vi "beam cup control - old.vi"() -> ()   [LabVIEW 2016, in "Top Level.lvlib"]
doc: "This vi is used to control the cups and apertures in the ams beamline."
uses:
  Top Level.lvlib
panel:
  in  "Which Beamline":string(combo)="R45"
  out "R45 detector cup":string="OUT"
  out "R45 detector aperture":string="IN"
  out "R45 switch image cup":string="IN"
  out "R45 switch aperture":string="OUT"
  in  "R30 detector ap":bool=TRUE
  out "R30 detector aperture":string="IN"
  out "R30 Detector cup rd":string="OUT"
  out "R30 switch aperture":string="IN"
  in  "R30 Image ap":bool=TRUE
  out "R30 switch image cup":string="OUT"
  out "analyze image cup rd":string="OUT"
  out "tank exit cup  rd":string="OUT"
  out "tank entrance cup  rd":string="OUT"
  out "low energy cup":string="OUT"
  out "injector image aperture":string="IN"
  out "injector cup":string="OUT"
  in  "r45 det cup":bool
  in  "R45  det ap":bool
  in  "r45 switch image cup":bool=TRUE
  in  "R45 #1 ap":bool
  out "Terminal Voltage":dbl=8.333384070396422 format="%#_4g"
  in  "R30 det cup":bool
  in  "Switch magnet cup":bool
  in  "Analyze image cup":bool
  in  "Tank exit cup":bool
  in  "Tank Entrance cup":bool
  in  "Low end waist  cup":bool=TRUE
  in  "Low end waist ap":bool
  in  "INJ Image ap":bool
  in  "Inj Image cup":bool
  out "date/time string":string="3/16/2012  11:07 AM"
  out "Error out":errorcluster
  in  "stop":bool
  # "Faraday cup Controls"
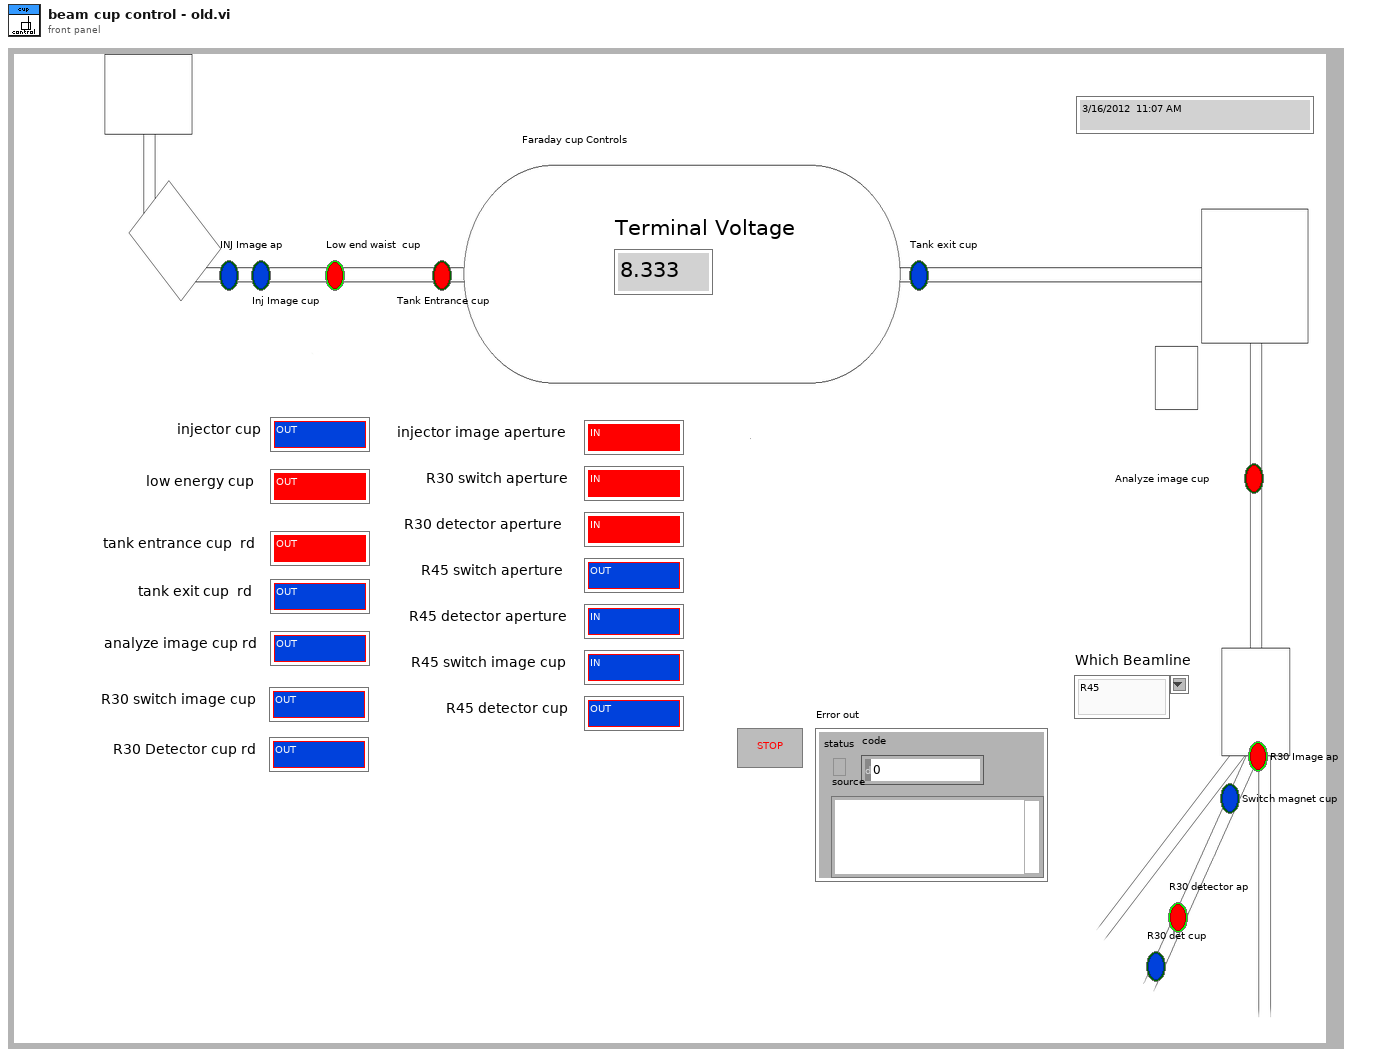
[diagram p1: front panel]
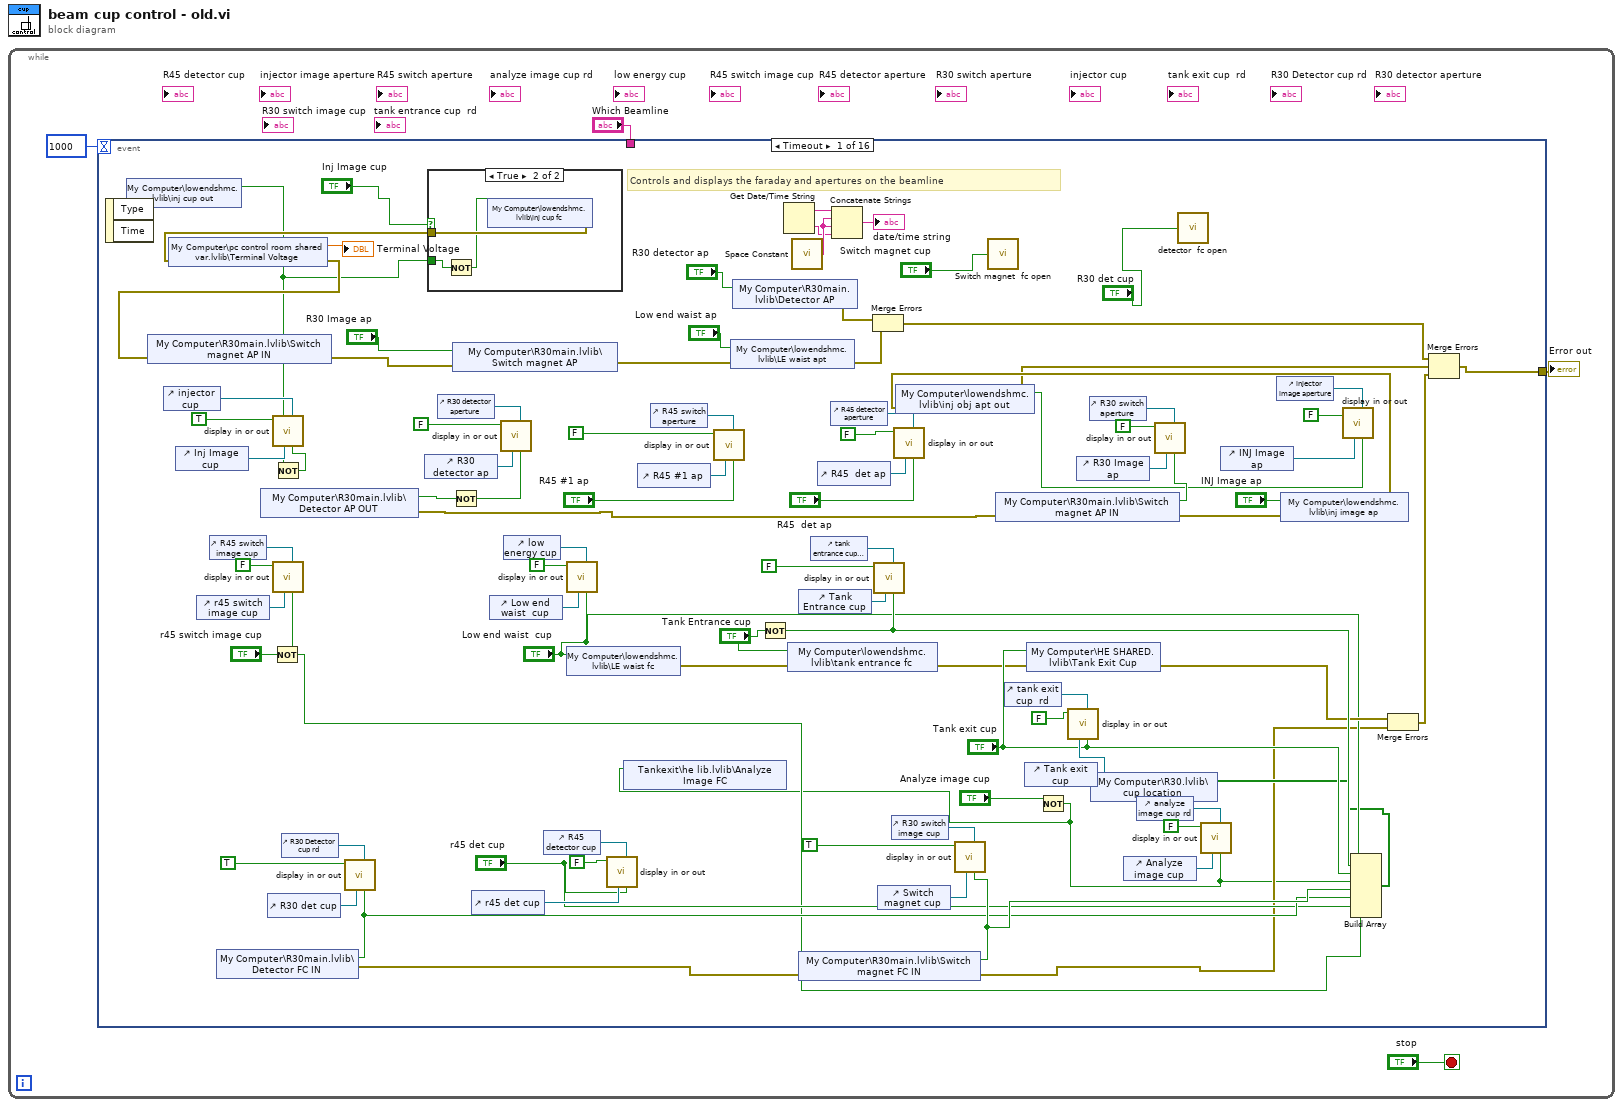
[diagram p0: block diagram]
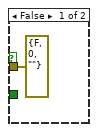
[diagram p2: hidden frame]
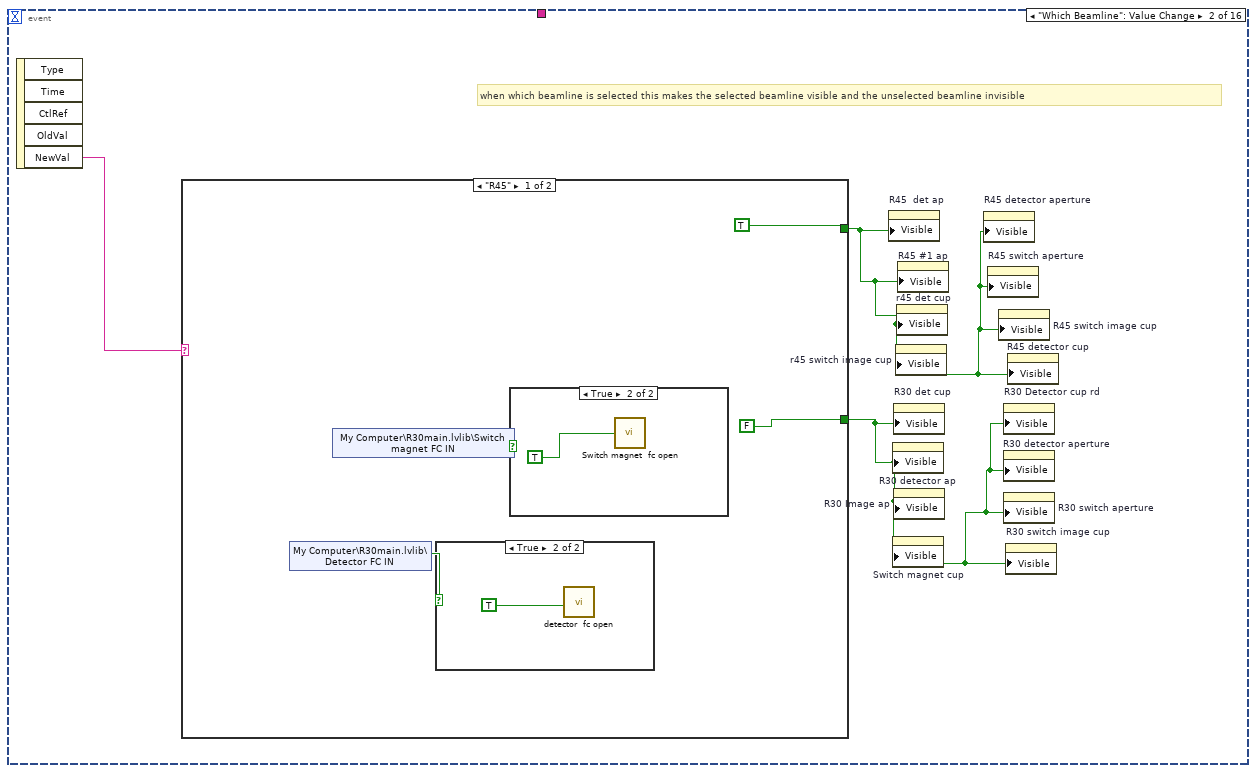
[diagram p3: hidden frame]
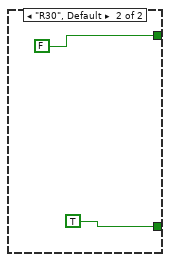
[diagram p6: hidden frame]
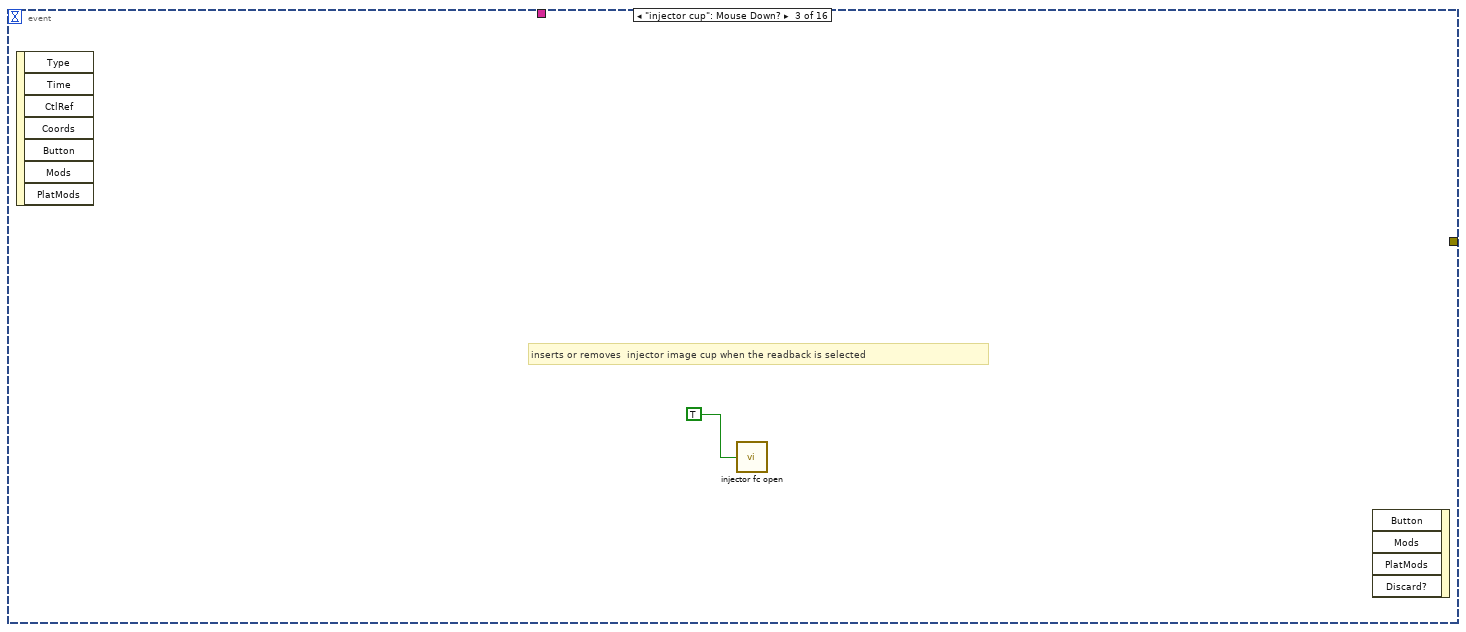
[diagram p7: hidden frame]
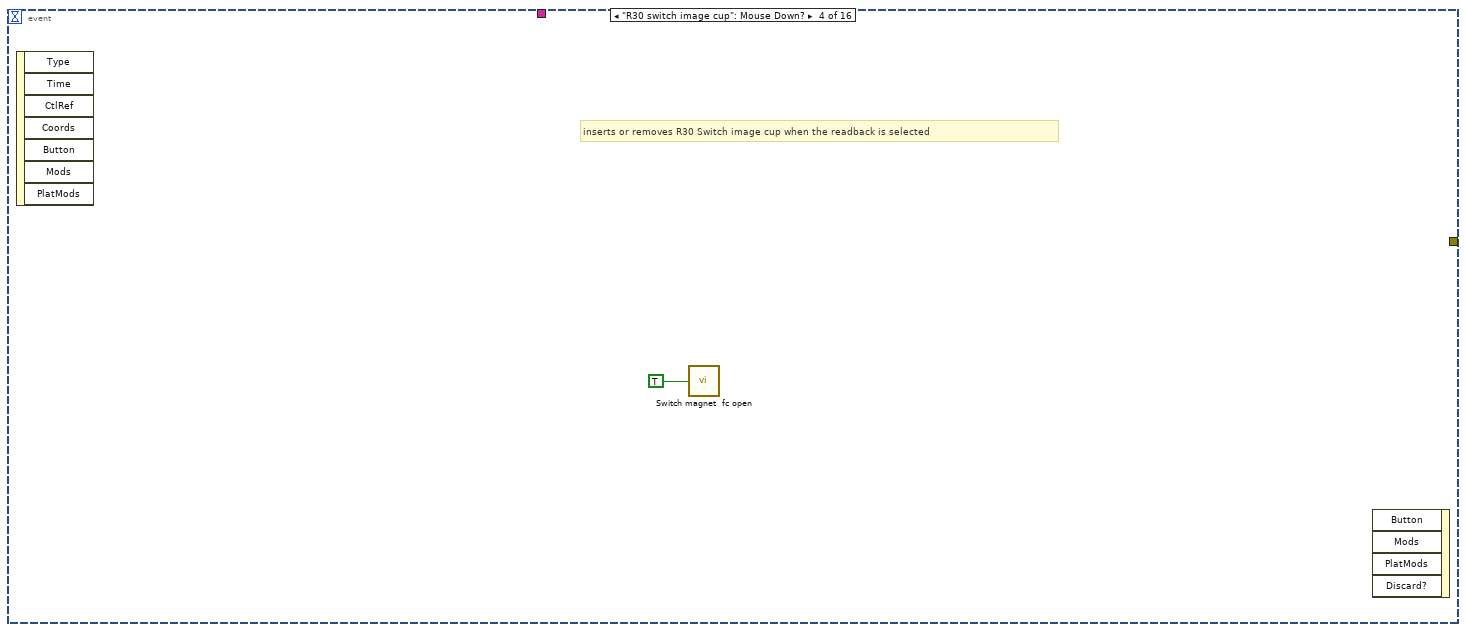
[diagram p8: hidden frame]
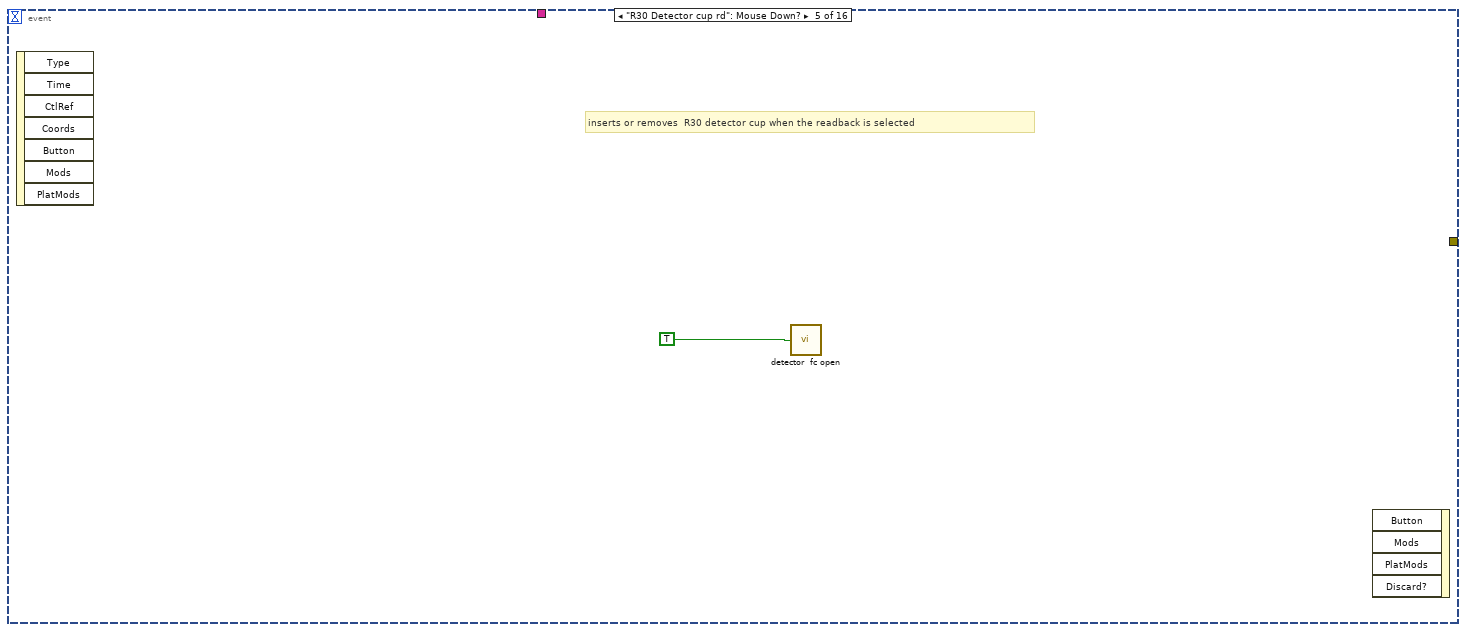
[diagram p9: hidden frame]
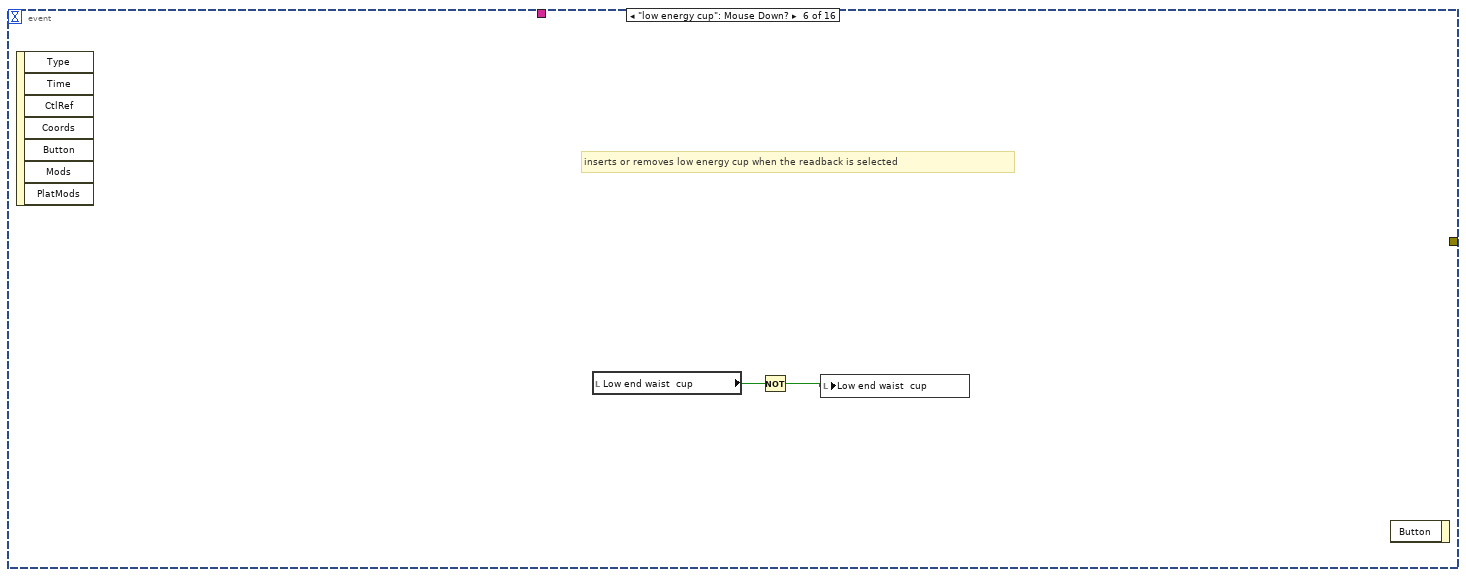
[diagram p10: hidden frame]
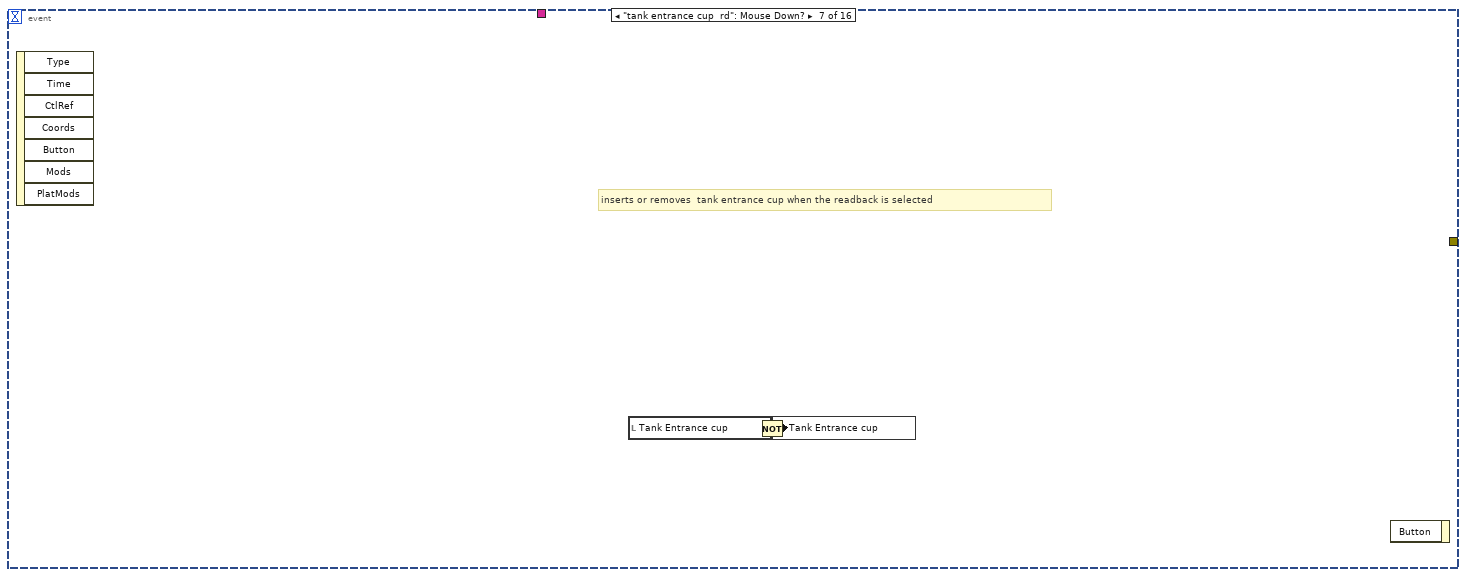
[diagram p11: hidden frame]
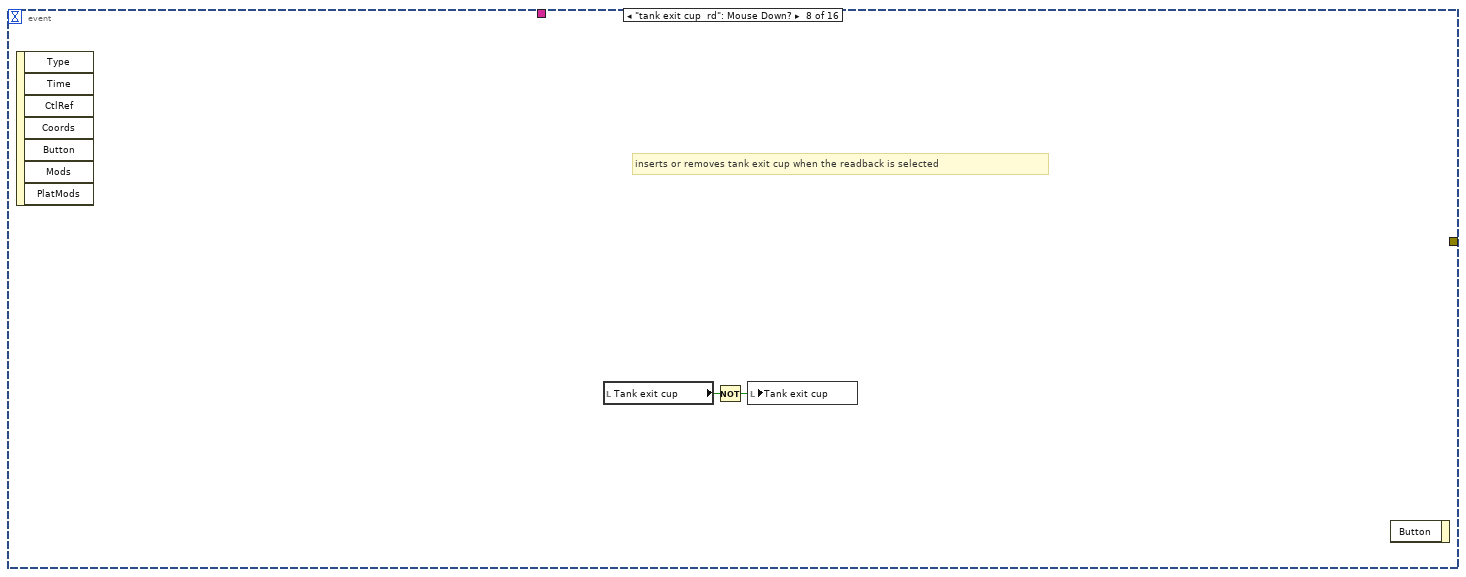
[diagram p12: hidden frame]
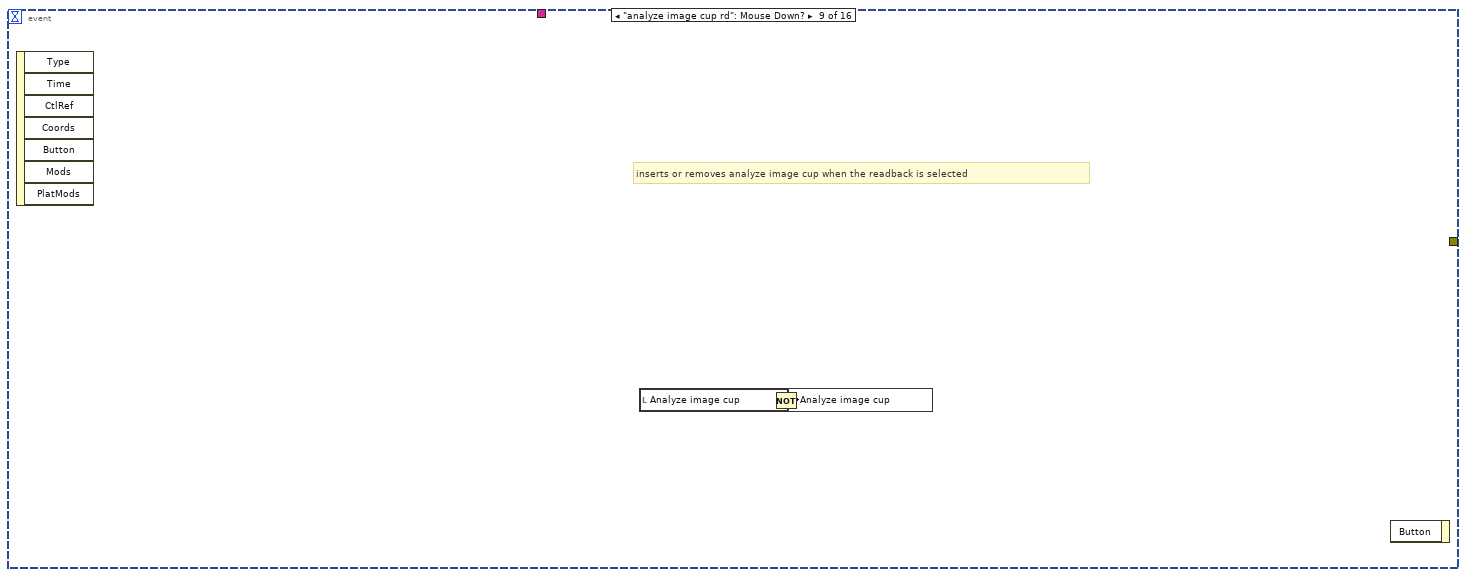
[diagram p13: hidden frame]
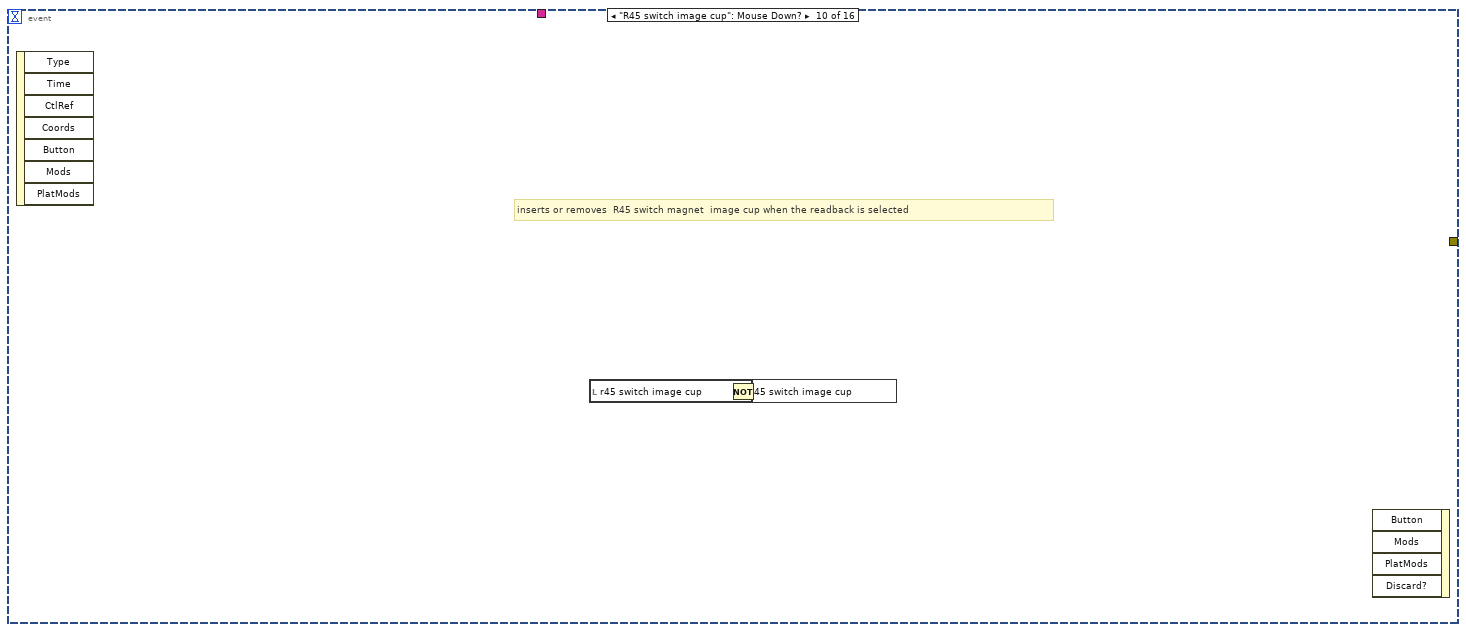
[diagram p14: hidden frame]
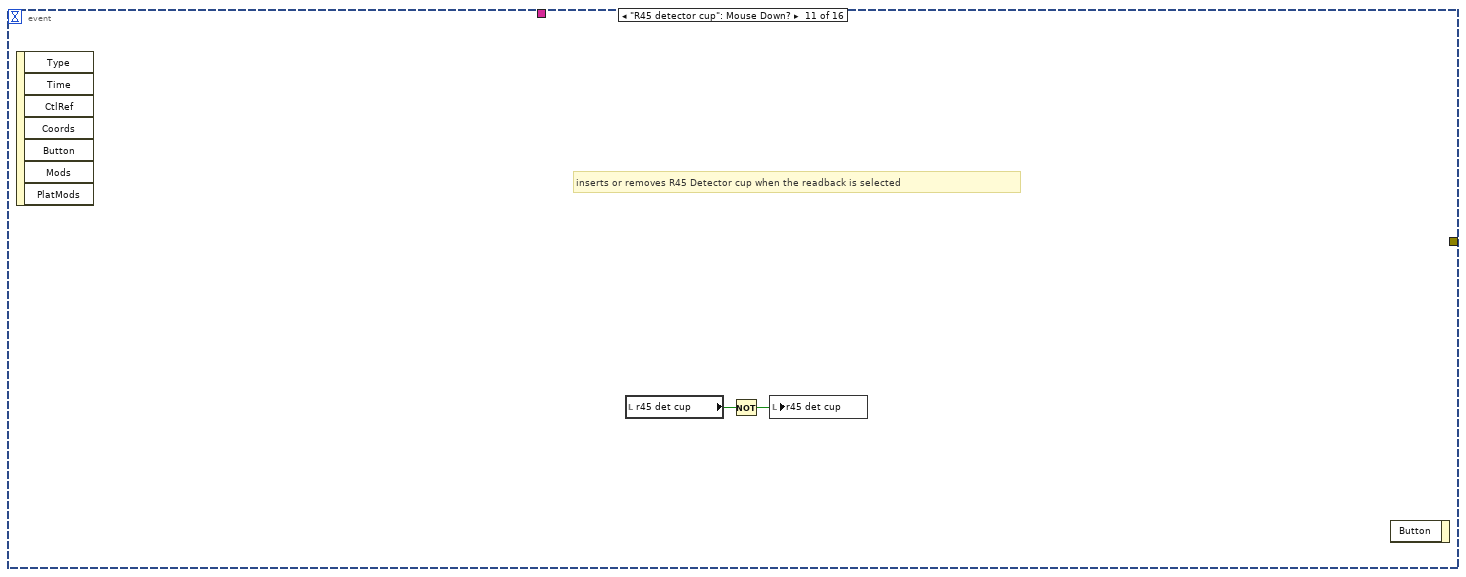
[diagram p15: hidden frame]
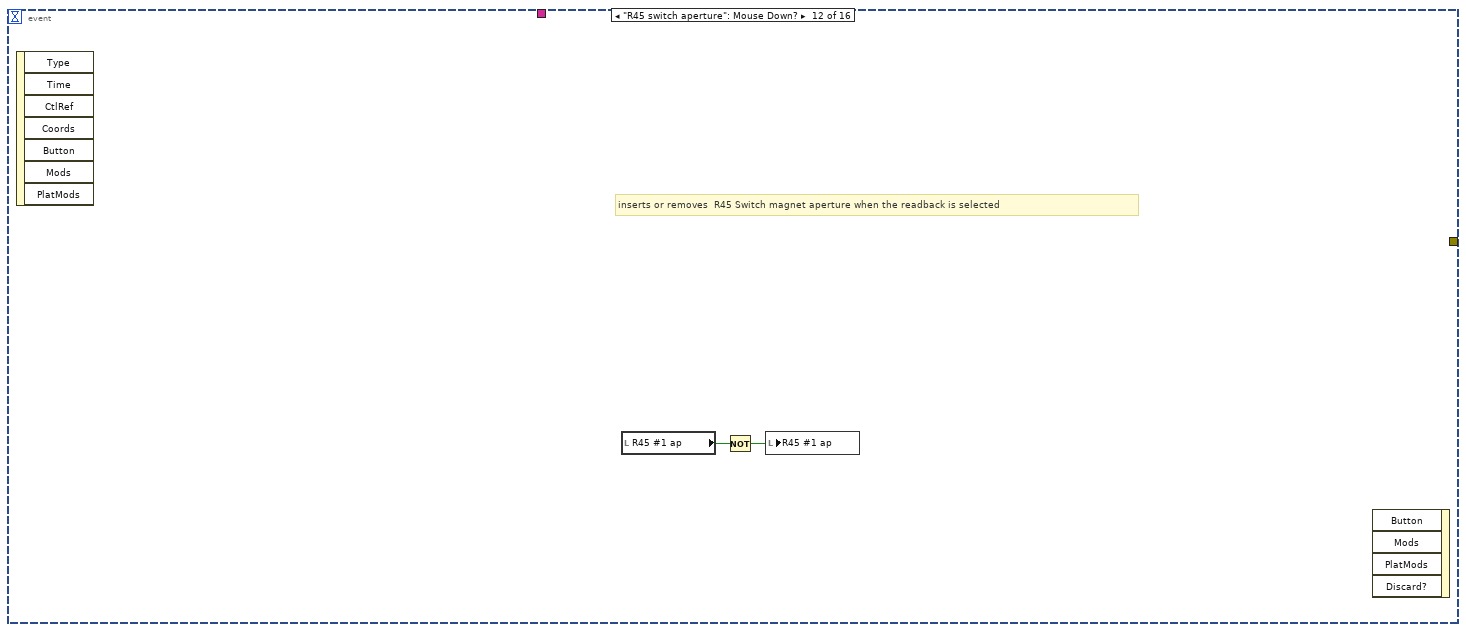
[diagram p16: hidden frame]
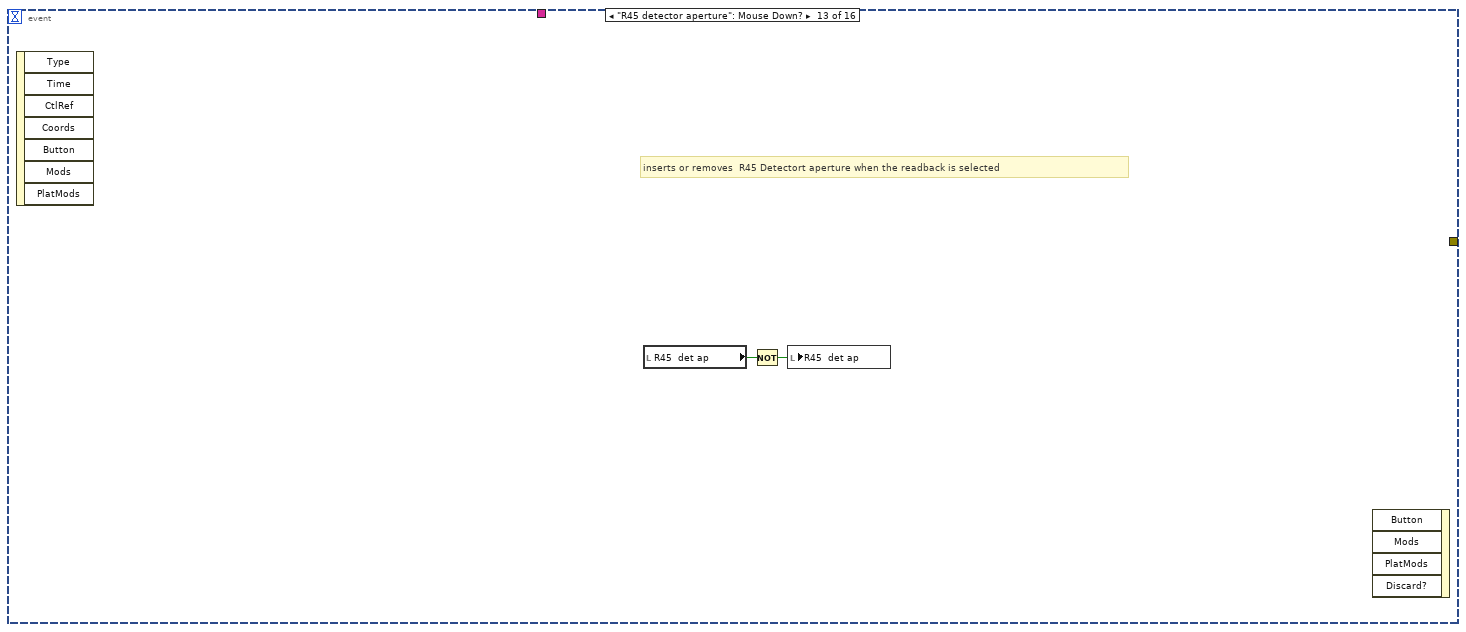
[diagram p17: hidden frame]
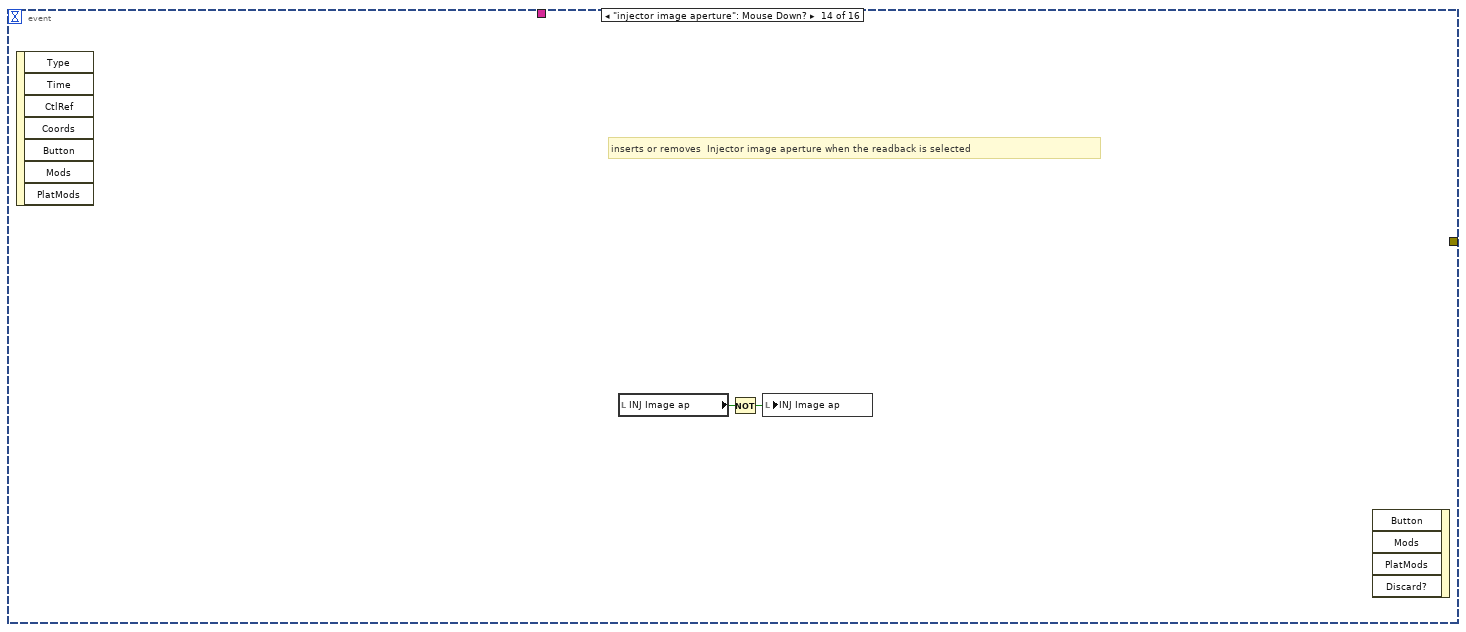
[diagram p18: hidden frame]
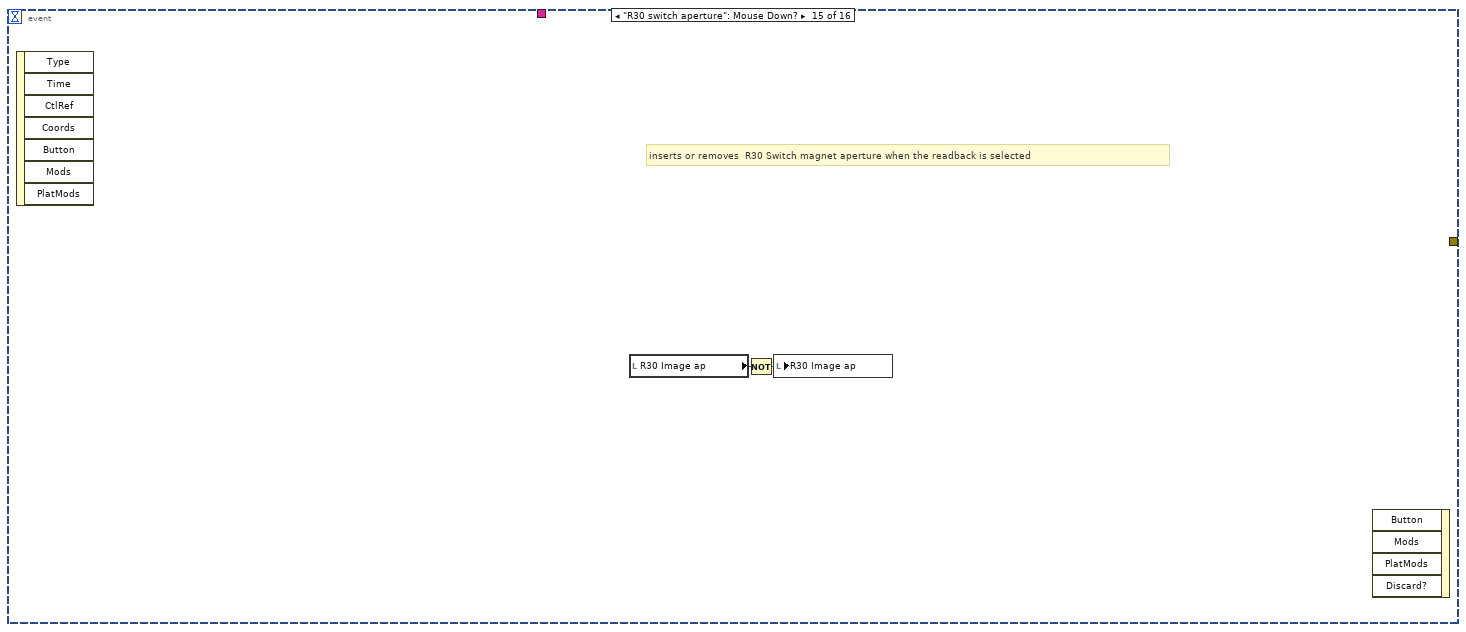
[diagram p19: hidden frame]
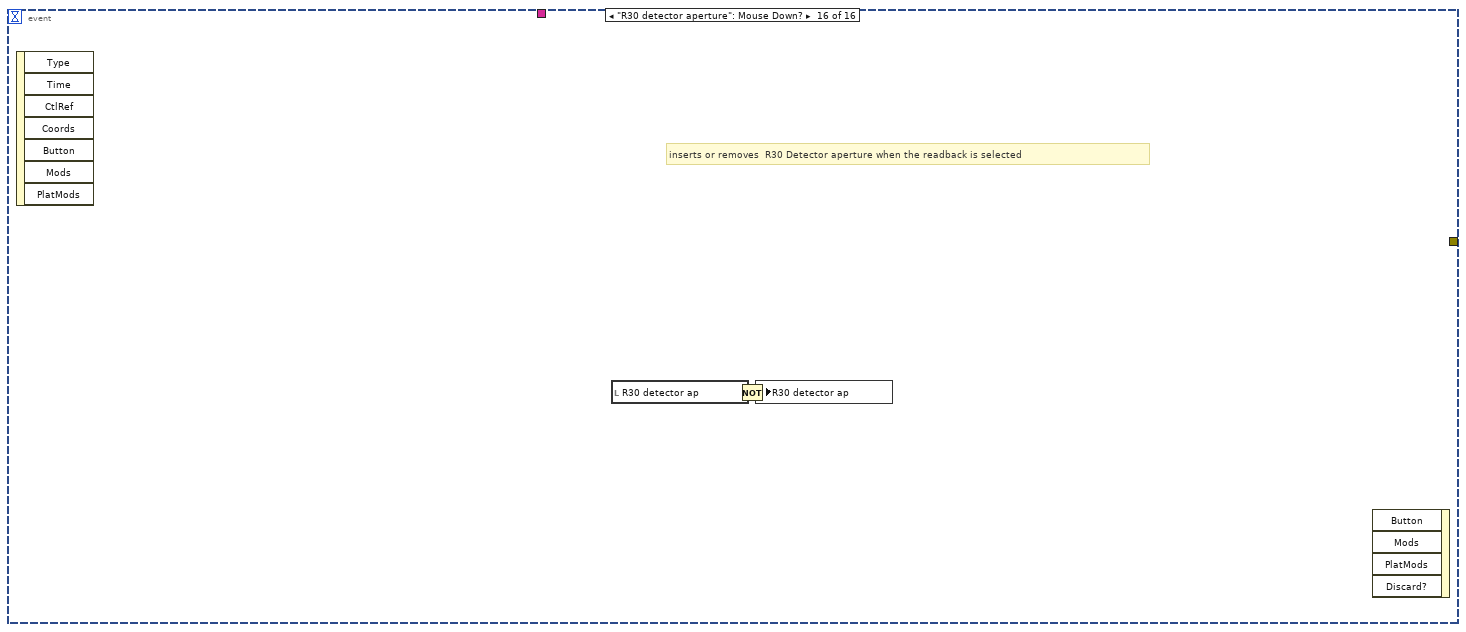
[diagram p20: hidden frame]
diagram:
  n1 = while {
    stop <- "stop" stop-if-true
    n2 = event shown="[0] Timeout" {
      selector: _ -> [_ _ _ _ _ _ _ _ _ _ _ _ _ _ _ _]
      dyn-events: _ -> [_ _ _ _ _ _ _ _ _ _ _ _ _ _ _ _]
      timeout: 1000 -> [_ _ _ _ _ _ _ _ _ _ _ _ _ _ _ _]
      tunnel: [w24 _ _ _ _ _ _ _ _ _ _ _ _ _ _ _] -> w2
      tunnel: "Which Beamline" -> [_ _ _ _ _ _ _ _ _ _ _ _ _ _ _ _]
      event Timeout {
        # "Controls and displays the faraday and apertures on the beamline"
        n3 = event-data() -> ()  [unwired: 1 in, 2 out]
        n4 = shared-variable "My Computer\\lowendshmc.lvlib\\inj cup out"() -> (w6:bool)  [unwired: 1 in, 1 out]
        n5 = control-ref of="injector cup"() -> (w92:refnum<vi>)
        n6 = control-ref of="Inj Image cup"() -> (w91:refnum<vi>)
        n7 = control-ref of="r45 switch image cup"() -> (w50:refnum<vi>)
        n8 = control-ref of="R45 switch image cup"() -> (w51:refnum<vi>)
        n9 = shared-variable "My Computer\\R30main.lvlib\\Detector FC IN"() -> (w62:bool, error out=w19:errorcluster)  [unwired: 1 in]
        n10 = shared-variable "My Computer\\R30main.lvlib\\Detector AP OUT"() -> (w57:bool, error out=w20:errorcluster)  [unwired: 1 in]
        n11 = control-ref of="R30 det cup"() -> (w64:refnum<vi>)
        n12 = Not(x="r45 switch image cup") -> (.not. x?=w15:bool)
        n13 = Not(x=w6) -> (.not. x?=w9:bool)
        n14 = call "display in or out.vi"("device in beam?"=w9, "in or out display Refnum"=w92, "device control Refnum"=w91, "use color control"=TRUE) -> ()  [unwired: 7 in, 1 out]
        n15 = call "display in or out.vi"("device in beam?"=w15, "in or out display Refnum"=w51, "device control Refnum"=w50, "use color control"=FALSE) -> ()  [unwired: 7 in, 1 out]
        n16 = control-ref of="R30 Detector cup rd"() -> (w65:refnum<vi>)
        n17 = call "display in or out.vi"("device in beam?"=w62, "in or out display Refnum"=w65, "device control Refnum"=w64, "use color control"=TRUE) -> ()  [unwired: 7 in, 1 out]
        n18 = control-ref of="R30 detector ap"() -> (w60:refnum<vi>)
        n19 = case shown="True" "Inj Image cup" {
          tunnel: [errorcluster {"status"=FALSE, "code"=0, "source"=""} ("error IO") w100] -> w11
          tunnel: w6 -> [_ w99]
          frame False {
          }
          frame True {
            n20 = Not(x=w99) -> (.not. x?=w98:bool)
            n21 = shared-variable "My Computer\\lowendshmc.lvlib\\inj cup fc"(w98) -> (error out=w100:errorcluster)  [unwired: 1 in]
          }
        }
        n22 = shared-variable "My Computer\\pc control room shared var.lvlib\\Terminal Voltage"(error in=w11) -> (→"Terminal Voltage":dbl, error out=w17:errorcluster)
        n23 = shared-variable "My Computer\\R30main.lvlib\\Switch magnet AP IN"(error in=w17) -> (error out=w37:errorcluster)  [unwired: 1 out]
        n24 = control-ref of="R30 detector aperture"() -> (w59:refnum<vi>)
        n25 = Not(x=w57) -> (.not. x?=w56:bool)
        n26 = shared-variable "My Computer\\R30main.lvlib\\Switch magnet AP"("R30 Image ap", error in=w37) -> (error out=w26:errorcluster)
        n27 = control-ref of="r45 det cup"() -> (w43:refnum<vi>)
        n28 = control-ref of="Low end waist  cup"() -> (w85:refnum<vi>)
        n29 = call "display in or out.vi"("device in beam?"=w56, "in or out display Refnum"=w59, "device control Refnum"=w60, "use color control"=FALSE) -> ()  [unwired: 7 in, 1 out]
        n30 = control-ref of="low energy cup"() -> (w84:refnum<vi>)
        n31 = control-ref of="R45 detector cup"() -> (w42:refnum<vi>)
        n32 = call "display in or out.vi"("device in beam?"="Low end waist  cup", "in or out display Refnum"=w84, "device control Refnum"=w85, "use color control"=FALSE) -> ()  [unwired: 7 in, 1 out]
        n33 = shared-variable "My Computer\\lowendshmc.lvlib\\LE waist fc"("Low end waist  cup") -> (error out=w35:errorcluster)  [unwired: 1 in]
        n34 = call "display in or out.vi"("device in beam?"="r45 det cup", "in or out display Refnum"=w42, "device control Refnum"=w43, "use color control"=FALSE) -> ()  [unwired: 7 in, 1 out]
        n35 = control-ref of="R45 #1 ap"() -> (w54:refnum<vi>)
        n36 = control-ref of="R45 switch aperture"() -> (w53:refnum<vi>)
        n37 = call "display in or out.vi"("device in beam?"="R45 #1 ap", "in or out display Refnum"=w53, "device control Refnum"=w54, "use color control"=FALSE) -> ()  [unwired: 7 in, 1 out]
        n38 = shared-variable "My Computer\\lowendshmc.lvlib\\LE waist apt"("Low end waist ap", error in=w26) -> (error out=w30:errorcluster)
        n39 = shared-variable "My Computer\\R30main.lvlib\\Detector AP"("R30 detector ap") -> (error out=w31:errorcluster)  [unwired: 1 in]
        n40 = Not(x="Tank Entrance cup") -> (.not. x?=w33:bool)
        n41 = Get Date/Time String() -> (date string=w96:string, time string=w93:string)  [unwired: 3 in]
        n42 = shared-variable "My Computer\\lowendshmc.lvlib\\tank entrance fc"("Tank Entrance cup", error in=w35) -> (error out=w34:errorcluster)
        n43 = call <vilib>:"Space Constant.vi"() -> ("String"=w94:string)
        n44 = control-ref of="Tank Entrance cup"() -> (w82:refnum<vi>)
        n45 = shared-variable "My Computer\\R30main.lvlib\\Switch magnet FC IN"(error in=w19) -> (w69:bool, error out=w8:errorcluster)
        n46 = control-ref of="tank entrance cup  rd"() -> (w83:refnum<vi>)
        n47 = control-ref of="R45  det ap"() -> (w47:refnum<vi>)
        n48 = control-ref of="R45 detector aperture"() -> (w48:refnum<vi>)
        n49 = Concatenate Strings(w96, w94, w94, w93) -> (→"date/time string":string)
        n50 = Merge Errors(w31, w30) -> (w29:errorcluster)
        n51 = call "display in or out.vi"("device in beam?"=w33, "in or out display Refnum"=w83, "device control Refnum"=w82, "use color control"=FALSE) -> ()  [unwired: 7 in, 1 out]
        n52 = control-ref of="Switch magnet cup"() -> (w71:refnum<vi>)
        n53 = control-ref of="R30 switch image cup"() -> (w70:refnum<vi>)
        n54 = call "display in or out.vi"("device in beam?"="R45  det ap", "in or out display Refnum"=w48, "device control Refnum"=w47, "use color control"=FALSE) -> ()  [unwired: 7 in, 1 out]
        n55 = call "display in or out.vi"("device in beam?"=w69, "in or out display Refnum"=w70, "device control Refnum"=w71, "use color control"=TRUE) -> ()  [unwired: 7 in, 1 out]
        n56 = call "Switch magnet  fc open.vi"("Faraday cup"="Switch magnet cup") -> ()
        n57 = shared-variable "My Computer\\R30main.lvlib\\Switch magnet AP IN"(error in=w20) -> (w58:bool, error out=w36:errorcluster)
        n58 = control-ref of="tank exit cup  rd"() -> (w77:refnum<vi>)
        n59 = control-ref of="Tank exit cup"() -> (w78:refnum<vi>)
        n60 = shared-variable "My Computer\\HE SHARED.lvlib\\Tank Exit Cup"("Tank exit cup", error in=w34) -> (error out=w32:errorcluster)
        n61 = Not(x="Analyze image cup") -> (.not. x?=w7:bool)
        n62 = shared-variable "Tankexit\\he lib.lvlib\\Analyze Image FC"(w7) -> ()  [unwired: 1 in, 1 out]
        n63 = call "display in or out.vi"("device in beam?"="Tank exit cup", "in or out display Refnum"=w77, "device control Refnum"=w78, "use color control"=FALSE) -> ()  [unwired: 7 in, 1 out]
        n64 = control-ref of="R30 Image ap"() -> (w67:refnum<vi>)
        n65 = control-ref of="R30 switch aperture"() -> (w68:refnum<vi>)
        n66 = control-ref of="Analyze image cup"() -> (w74:refnum<vi>)
        n67 = control-ref of="analyze image cup rd"() -> (w75:refnum<vi>)
        n68 = call "display in or out.vi"("device in beam?"=w58, "in or out display Refnum"=w68, "device control Refnum"=w67, "use color control"=FALSE) -> ()  [unwired: 7 in, 1 out]
        n69 = call "detector  fc open.vi"("Faraday cup"="R30 det cup") -> ()
        n70 = call "display in or out.vi"("device in beam?"=w7, "in or out display Refnum"=w75, "device control Refnum"=w74, "use color control"=FALSE) -> ()  [unwired: 7 in, 1 out]
        n71 = control-ref of="INJ Image ap"() -> (w89:refnum<vi>)
        n72 = control-ref of="injector image aperture"() -> (w90:refnum<vi>)
        n73 = shared-variable "My Computer\\lowendshmc.lvlib\\inj image ap"("INJ Image ap", error in=w36) -> (error out=w13:errorcluster)
        n74 = shared-variable "My Computer\\lowendshmc.lvlib\\inj obj apt out"(error in=w13) -> (w14:bool, error out=w12:errorcluster)
        n75 = call "display in or out.vi"("device in beam?"=w14, "in or out display Refnum"=w90, "device control Refnum"=w89, "use color control"=FALSE) -> ()  [unwired: 7 in, 1 out]
        n76 = Build Array("Low end waist  cup", w33, "Tank exit cup", w7, w69, w62, w15, "r45 det cup") -> (w16:bool[])
        n77 = shared-variable "My Computer\\R30.lvlib\\cup location"(w16) -> ()  [unwired: 1 in, 1 out]
        n78 = Merge Errors(w32, w8) -> (w28:errorcluster)
        n79 = Merge Errors(w29, w12, w28) -> (w24:errorcluster)
      }
      event "Which Beamline": Value Change {
        # "when which beamline is selected this makes the selected beamline visible and the unselected beamline invisible"
        n80 = event-data() -> ("NewVal"=w103:string)  [unwired: 1 in, 4 out]
        n81 = case shown="\"R45\"" w103 {
          tunnel: [TRUE ("Visible") FALSE ("Visible")] -> w101
          tunnel: [FALSE ("Visible") TRUE ("Visible")] -> w102
          frame "R45" {
            n82 = shared-variable "My Computer\\R30main.lvlib\\Detector FC IN"() -> (w104:bool)  [unwired: 1 in, 1 out]
            n83 = shared-variable "My Computer\\R30main.lvlib\\Switch magnet FC IN"() -> (w105:bool)  [unwired: 1 in, 1 out]
            n84 = case shown="True" w104 {
              frame False {
              }
              frame True {
                n85 = call "detector  fc open.vi"("Faraday cup"=TRUE ("inj cup fc")) -> ()
              }
            }
            n86 = case shown="True" w105 {
              frame False {
              }
              frame True {
                n87 = call "Switch magnet  fc open.vi"("Faraday cup"=TRUE ("inj cup fc")) -> ()
              }
            }
          }
          frame "R30", Default {
          }
        }
        n88 = property on="R45  det ap" class="Bool (strict)"("Visible"=w101) -> ()  [unwired: 2 in, 2 out]
        n89 = property on="R30 detector ap" class="Bool (strict)"("Visible"=w102) -> ()  [unwired: 2 in, 2 out]
        n90 = property on="Switch magnet cup" class="Bool"("Visible"=w102) -> ()  [unwired: 2 in, 2 out]
        n91 = property on="R30 det cup" class="Bool"("Visible"=w102) -> ()  [unwired: 2 in, 2 out]
        n92 = property on="R30 Image ap" class="Bool (strict)"("Visible"=w102) -> ()  [unwired: 2 in, 2 out]
        n93 = property on="r45 switch image cup" class="Bool (strict)"("Visible"=w101) -> ()  [unwired: 2 in, 2 out]
        n94 = property on="r45 det cup" class="Bool (strict)"("Visible"=w101) -> ()  [unwired: 2 in, 2 out]
        n95 = property on="R45 #1 ap" class="Bool (strict)"("Visible"=w101) -> ()  [unwired: 2 in, 2 out]
        n96 = property on="R45 detector aperture" class="Str"("Visible"=w101) -> ()  [unwired: 2 in, 2 out]
        n97 = property on="R45 switch aperture" class="Str"("Visible"=w101) -> ()  [unwired: 2 in, 2 out]
        n98 = property on="R45 switch image cup" class="Str"("Visible"=w101) -> ()  [unwired: 2 in, 2 out]
        n99 = property on="R30 Detector cup rd" class="Str"("Visible"=w102) -> ()  [unwired: 2 in, 2 out]
        n100 = property on="R30 detector aperture" class="Str"("Visible"=w102) -> ()  [unwired: 2 in, 2 out]
        n101 = property on="R30 switch aperture" class="Str"("Visible"=w102) -> ()  [unwired: 2 in, 2 out]
        n102 = property on="R30 switch image cup" class="Str"("Visible"=w102) -> ()  [unwired: 2 in, 2 out]
        n103 = property on="R45 detector cup" class="Str"("Visible"=w101) -> ()  [unwired: 2 in, 2 out]
      }
      event "injector cup": Mouse Down? {
        # "inserts or removes  injector image cup when the readback is selected"
        n104 = event-data() -> ()  [unwired: 1 in, 7 out]
        n105 = call "injector fc open.vi"("Faraday cup"=TRUE ("inj cup fc")) -> ()
        n106 = event-data() -> ()  [unwired: 5 in, 1 out]
      }
      event "R30 switch image cup": Mouse Down? {
        # "inserts or removes R30 Switch image cup when the readback is selected"
        n107 = event-data() -> ()  [unwired: 1 in, 7 out]
        n108 = call "Switch magnet  fc open.vi"("Faraday cup"=TRUE ("inj cup fc")) -> ()
        n109 = event-data() -> ()  [unwired: 5 in, 1 out]
      }
      event "R30 Detector cup rd": Mouse Down? {
        # "inserts or removes  R30 detector cup when the readback is selected"
        n110 = event-data() -> ()  [unwired: 1 in, 7 out]
        n111 = call "detector  fc open.vi"("Faraday cup"=TRUE ("inj cup fc")) -> ()
        n112 = event-data() -> ()  [unwired: 5 in, 1 out]
      }
      event "low energy cup": Mouse Down? {
        # "inserts or removes low energy cup when the readback is selected"
        n113 = event-data() -> ()  [unwired: 1 in, 7 out]
        n114 = local read "Low end waist  cup"() -> (w116:bool)
        n115 = Not(x=w116) -> (.not. x?=w115:bool)
        n116 = local write "Low end waist  cup"(w115) -> ()
        n117 = event-data() -> ()  [unwired: 2 in, 1 out]
      }
      event "tank entrance cup  rd": Mouse Down? {
        # "inserts or removes  tank entrance cup when the readback is selected"
        n118 = event-data() -> ()  [unwired: 1 in, 7 out]
        n119 = local read "Tank Entrance cup"() -> (w118:bool)
        n120 = Not(x=w118) -> (.not. x?=w117:bool)
        n121 = local write "Tank Entrance cup"(w117) -> ()
        n122 = event-data() -> ()  [unwired: 2 in, 1 out]
      }
      event "tank exit cup  rd": Mouse Down? {
        # "inserts or removes tank exit cup when the readback is selected"
        n123 = event-data() -> ()  [unwired: 1 in, 7 out]
        n124 = local read "Tank exit cup"() -> (w120:bool)
        n125 = Not(x=w120) -> (.not. x?=w119:bool)
        n126 = local write "Tank exit cup"(w119) -> ()
        n127 = event-data() -> ()  [unwired: 2 in, 1 out]
      }
      event "analyze image cup rd": Mouse Down? {
        # "inserts or removes analyze image cup when the readback is selected"
        n128 = event-data() -> ()  [unwired: 1 in, 7 out]
        n129 = local read "Analyze image cup"() -> (w122:bool)
        n130 = Not(x=w122) -> (.not. x?=w121:bool)
        n131 = local write "Analyze image cup"(w121) -> ()
        n132 = event-data() -> ()  [unwired: 2 in, 1 out]
      }
      event "R45 switch image cup": Mouse Down? {
        # "inserts or removes  R45 switch magnet  image cup when the readback is selected"
        n133 = event-data() -> ()  [unwired: 1 in, 7 out]
        n134 = local read "r45 switch image cup"() -> (w124:bool)
        n135 = Not(x=w124) -> (.not. x?=w123:bool)
        n136 = local write "r45 switch image cup"(w123) -> ()
        n137 = event-data() -> ()  [unwired: 5 in, 1 out]
      }
      event "R45 detector cup": Mouse Down? {
        # "inserts or removes R45 Detector cup when the readback is selected"
        n138 = event-data() -> ()  [unwired: 1 in, 7 out]
        n139 = local read "r45 det cup"() -> (w126:bool)
        n140 = Not(x=w126) -> (.not. x?=w125:bool)
        n141 = local write "r45 det cup"(w125) -> ()
        n142 = event-data() -> ()  [unwired: 2 in, 1 out]
      }
      event "R45 switch aperture": Mouse Down? {
        # "inserts or removes  R45 Switch magnet aperture when the readback is selected"
        n143 = event-data() -> ()  [unwired: 1 in, 7 out]
        n144 = local read "R45 #1 ap"() -> (w128:bool)
        n145 = Not(x=w128) -> (.not. x?=w127:bool)
        n146 = local write "R45 #1 ap"(w127) -> ()
        n147 = event-data() -> ()  [unwired: 5 in, 1 out]
      }
      event "R45 detector aperture": Mouse Down? {
        # "inserts or removes  R45 Detectort aperture when the readback is selected"
        n148 = event-data() -> ()  [unwired: 1 in, 7 out]
        n149 = local read "R45  det ap"() -> (w130:bool)
        n150 = Not(x=w130) -> (.not. x?=w129:bool)
        n151 = local write "R45  det ap"(w129) -> ()
        n152 = event-data() -> ()  [unwired: 5 in, 1 out]
      }
      event "injector image aperture": Mouse Down? {
        # "inserts or removes  Injector image aperture when the readback is selected"
        n153 = event-data() -> ()  [unwired: 1 in, 7 out]
        n154 = local read "INJ Image ap"() -> (w132:bool)
        n155 = Not(x=w132) -> (.not. x?=w131:bool)
        n156 = local write "INJ Image ap"(w131) -> ()
        n157 = event-data() -> ()  [unwired: 5 in, 1 out]
      }
      event "R30 switch aperture": Mouse Down? {
        # "inserts or removes  R30 Switch magnet aperture when the readback is selected"
        n158 = event-data() -> ()  [unwired: 1 in, 7 out]
        n159 = local read "R30 Image ap"() -> (w134:bool)
        n160 = Not(x=w134) -> (.not. x?=w133:bool)
        n161 = local write "R30 Image ap"(w133) -> ()
        n162 = event-data() -> ()  [unwired: 5 in, 1 out]
      }
      event "R30 detector aperture": Mouse Down? {
        # "inserts or removes  R30 Detector aperture when the readback is selected"
        n163 = event-data() -> ()  [unwired: 1 in, 7 out]
        n164 = local read "R30 detector ap"() -> (w136:bool)
        n165 = Not(x=w136) -> (.not. x?=w135:bool)
        n166 = local write "R30 detector ap"(w135) -> ()
        n167 = event-data() -> ()  [unwired: 5 in, 1 out]
      }
    }
    "Error out" <- w2
  }
